vi "Configure Single Channel Phase.vi"(6 "Phase Unwrap (T: Enable)":bool=TRUE, 7 "Amplitude Threshold (0)":dbl, 8 "error in (no error)":errorcluster, 9 "Input Type (0: Analog)":i32(ring) items=["Analog", "Digital"], 10 "Analyzer (0: A0)":i32(ring) items=["A0", "A1"], 11 "VISA resource name":refnum<visa-resource-name>) -> (0 "error out":errorcluster, 3 "VISA resource name out":refnum<visa-resource-name>)   [LabVIEW 2014, in "Stanford Research SR1.lvlib"]
doc: "Configures the attributes of the Single Channel Phase."
uses:
  Stanford Research SR1.lvlib
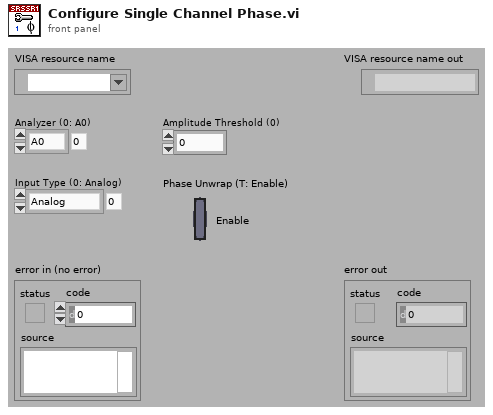
[diagram p1: front panel]
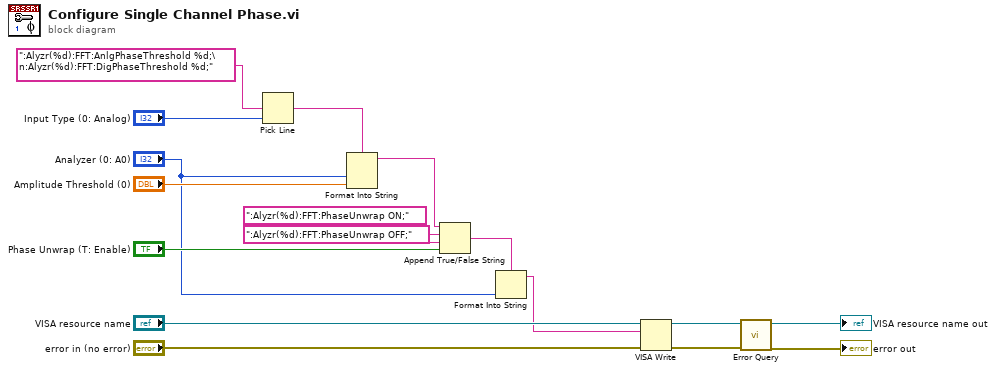
[diagram p0: block diagram]
diagram:
  n1 = Pick Line(multi-line string=":Alyzr(%d):FFT:AnlgPhaseThreshold %d;\n:Alyzr(%d):FFT:DigPhaseThreshold %d;", line index="Input Type (0: Analog)") -> (output string=w9:string)  [unwired: 1 in]
  n2 = Format Into String(format string=w9, "Analyzer (0: A0)", "Amplitude Threshold (0)") -> (resulting string=w1:string)  [unwired: 2 in, 1 out]
  n3 = Append True/False String(1:"Phase Unwrap (T: Enable)", 2:":Alyzr(%d):FFT:PhaseUnwrap OFF;" ("false string"), 3:":Alyzr(%d):FFT:PhaseUnwrap ON;" ("true string"), 4:w1) -> (0:w4:string)
  n4 = Format Into String(format string=w4, "Analyzer (0: A0)") -> (resulting string=w2:string)  [unwired: 2 in, 1 out]
  n5 = VISA Write(VISA resource name="VISA resource name", write buffer=w2, error in (no error)="error in (no error)") -> (VISA resource name out=w15:refnum<visa-resource-name>, error out=w14:errorcluster)  [unwired: 1 out]
  n6 = call "Error Query.vi"("error in (no error)"=w14, "VISA resource name"=w15) -> ("error out"=→"error out":errorcluster, "VISA resource name out"=→"VISA resource name out":refnum<visa-resource-name>)  [unwired: 6 in, 2 out]
